vi "snippet get main ui alias names.vi"() -> ()   [LabVIEW 2017]
uses:
  <vilib>/TELLC/CtrlRef/TD UI Control Label-IONames--cluster.ctl
  <vilib>/TELLC/CtrlRef/TD UI Control Label-Alias-IOName--cluster.ctl
  LV_Source/Application/DataTypes/MainUI CtrlRef AliasNames--enum.ctl
panel:
  in  "Ring":u16(ring)
  out "Array":string[](array[string])
  in  "AliasCtrlNames":T1
  in  "UI Control Label Associations":T2={"Controls"=[{"Label"="Application in", "Alias"="", "IOName"=""}, {"Label"="MainTabCtrl", "Alias"="", "IOName"=""}, {"Label"="MoveTowardFast", "Alias"="", "IOName"=""}, {"Label"="MoveToZero", "Alias"="", "IOName"=""}, {"Label"="MoveAwayFast", "Alias"="", "IOName"=""}, {"Label"="MoveToward", "Alias"="", "IOName"=""}, {"Label"="MoveAway", "Alias"="", "IOName"=""}, {"Label"="Safety OK", "Alias"="", "IOName"=""}, {"Label"="SystemError", "Alias"="", "IOName"=""}, {"Label"="Pos Err (cnts)", "Alias"="", "IOName"=""}, {"Label"="MotorPos(in)", "Alias"="", "IOName"=""}, {"Label"="StatusMsg", "Alias"="", "IOName"=""}, {"Label"="Weld Enable", "Alias"="", "IOName"=""}, {"Label"="JoggingTurntable", "Alias"="", "IOName"=""}, {"Label"="JogTurntable", "Alias"="", "IOName"=""}, {"Label"="SeqLoaded", "Alias"="", "IOName"=""}, {"Label"="SeqAborted", "Alias"="", "IOName"=""}, {"Label"="AbortSeq", "Alias"="", "IOName"=""}, {"Label"="MotorCtrlLoop Enable", "Alias"="", "IOName"=""}, {"Label"="Turntable Enable", "Alias"="", "IOName"=""}, {"Label"="SeqRunning", "Alias"="", "IOName"=""}, {"Label"="StartSeq", "Alias"="", "IOName"=""}, {"Label"="Sequence File", "Alias"="", "IOName"=""}, {"Label"="Tab Control", "Alias"="", "IOName"=""}, {"Label"="IgnoreMtrRspnsErr", "Alias"="", "IOName"=""}, {"Label"="AVC ConfigUtility", "Alias"="", "IOName"=""}, {"Label"="SamplingRate", "Alias"="", "IOName"=""}, {"Label"="NumSamples", "Alias"="", "IOName"=""}, {"Label"="UpdateDAQSettings", "Alias"="", "IOName"=""}, {"Label"="DAQ Rd & MtrSP Interval", "Alias"="", "IOName"=""}, {"Label"="WriteLogFile Interval", "Alias"="", "IOName"=""}, {"Label"="DAQDisplay Interval", "Alias"="", "IOName"=""}, {"Label"="DAQEnabled", "Alias"="", "IOName"=""}, {"Label"="DAQEnDis", "Alias"="", "IOName"=""}, {"Label"="LogEnabled", "Alias"="", "IOName"=""}, {"Label"="LogEnDis", "Alias"="", "IOName"=""}, {"Label"="TDMSEnabled", "Alias"="", "IOName"=""}, {"Label"="TDMSEnDis", "Alias"="", "IOName"=""}, {"Label"="PosCtlrSettings", "Alias"="", "IOName"=""}, {"Label"="MotorRspnsErr", "Alias"="", "IOName"=""}, {"Label"="TotalVgain", "Alias"="", "IOName"=""}, {"Label"="Motor SP", "Alias"="", "IOName"=""}, {"Label"="VoltageError", "Alias"="", "IOName"=""}, {"Label"="WeldTime", "Alias"="", "IOName"=""}, {"Label"="voltage fb", "Alias"="", "IOName"=""}, {"Label"="Current SP", "Alias"="", "IOName"=""}, {"Label"="Current fb", "Alias"="", "IOName"=""}, {"Label"="ProcessTime", "Alias"="", "IOName"=""}, {"Label"="AVC Lockout", "Alias"="", "IOName"=""}, {"Label"="In Range?", "Alias"="", "IOName"=""}, {"Label"="VspOffset", "Alias"="", "IOName"=""}, {"Label"="Volts and Current Chart", "Alias"="", "IOName"=""}, {"Label"="GraphEnable", "Alias"="", "IOName"=""}, {"Label"="DAQ Latency", "Alias"="", "IOName"=""}, {"Label"="MotorControlUI", "Alias"="", "IOName"=""}, {"Label"="SeqList", "Alias"="", "IOName"=""}, {"Label"="Step Comment", "Alias"="", "IOName"=""}, {"Label"="Turntable \nSpeed (RPM)", "Alias"="", "IOName"=""}, {"Label"="Process Complete", "Alias"="", "IOName"=""}, {"Label"="Weld Profile Graph", "Alias"="", "IOName"=""}, {"Label"="Weld Current Waveform Chart", "Alias"="", "IOName"=""}, {"Label"="Exit", "Alias"="", "IOName"=""}, {"Label"="LoadSeq", "Alias"="", "IOName"=""}, {"Label"="Exit2", "Alias"="", "IOName"=""}, {"Label"="Get DAQ Data", "Alias"="", "IOName"=""}, {"Label"="DAQ Data", "Alias"="", "IOName"=""}, {"Label"="time stamp", "Alias"="", "IOName"=""}, {"Label"="col 0", "Alias"="", "IOName"=""}, {"Label"="col 1", "Alias"="", "IOName"=""}, {"Label"="col 0 name", "Alias"="", "IOName"=""}, {"Label"="col 1 name", "Alias"="", "IOName"=""}, {"Label"="DI DAQ Data", "Alias"="", "IOName"=""}, {"Label"="Sequence Table", "Alias"="", "IOName"=""}, {"Label"="SeqSteps[]", "Alias"="", "IOName"=""}, {"Label"="SeqFileParams", "Alias"="", "IOName"=""}, {"Label"="Load Seq (debug)", "Alias"="", "IOName"=""}, {"Label"="LoadSeqStatus", "Alias"="", "IOName"=""}, {"Label"="SeqFilePathname", "Alias"="", "IOName"=""}, {"Label"="SeqExecStatus", "Alias"="", "IOName"=""}, {"Label"="LocalSMDirect EvData", "Alias"="", "IOName"=""}, {"Label"="AbortSeq - NonLatchingCtrl", "Alias"="", "IOName"=""}]}
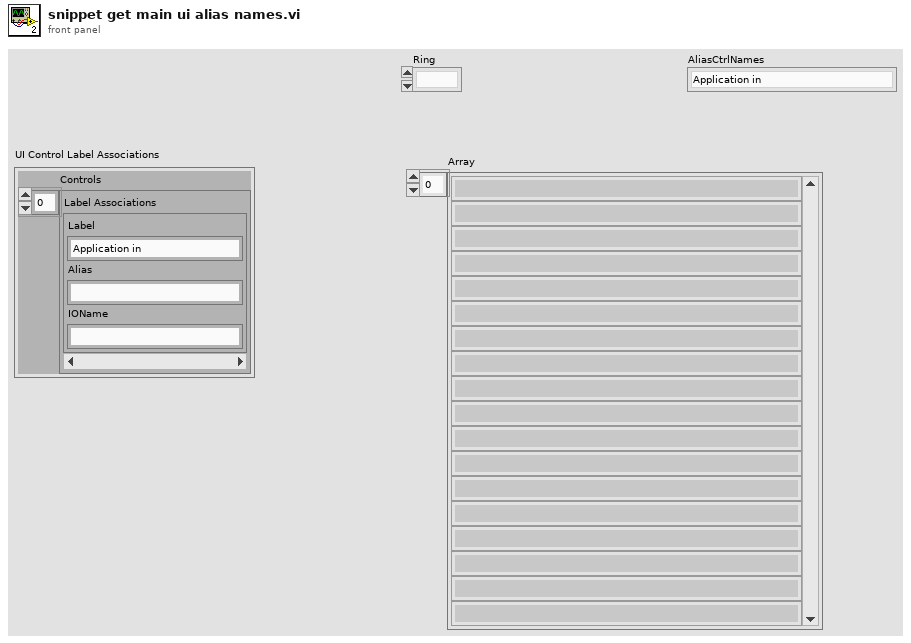
[diagram p1: front panel]
types:
  T1 = typedef "Application.lvclass/MainUI CtrlRef AliasNames--enum.ctl" = enum16{"Application in", "MainTabCtrl", "MoveTowardFast", "MoveToZero", "MoveAwayFast", "MoveToward", "MoveAway", "Safety OK", "SystemError", "Pos Err (cnts)", "MotorPos(in)", "StatusMsg", "Weld Enable", "JoggingTurntable", "JogTurntable", "SeqLoaded", "SeqAborted", "AbortSeq", "MotorCtrlLoop Enable", "Turntable Enable", "SeqRunning", "StartSeq", "Sequence File", "Tab Control", "IgnoreMtrRspnsErr", "AVC ConfigUtility", "SamplingRate", "NumSamples", "UpdateDAQSettings", "DAQ Rd & MtrSP Interval", "WriteLogFile Interval", "DAQDisplay Interval", "DAQEnabled", "DAQEnDis", "LogEnabled", "LogEnDis", "TDMSEnabled", "TDMSEnDis", "PosCtlrSettings", "MotorRspnsErr", "TotalVgain", "Motor SP", "VoltageError", "WeldTime", "voltage fb", "Current SP", "Current fb", "ProcessTime", "AVC Lockout", "In Range?", "VspOffset", "Volts and Current Chart", "GraphEnable", "DAQ Latency", "MotorControlUI", "SeqList", "Step Comment", "Turntable Speed (RPM)", "Process Complete", "Weld Profile Graph", "Weld Current Waveform Chart", "Exit", "LoadSeq", "Exit2", "Get DAQ Data", "DAQ Data", "time stamp", "col 0", "col 1", "col 0 name", "col 1 name", "DI DAQ Data", "Sequence Table", "SeqSteps[]", "SeqFileParams", "Load Seq (debug)", "LoadSeqStatus", "SeqFilePathname", "SeqExecStatus", "LocalSMDirect EvData", "AbortSeq - NonLatchingCtrl"}
  T2 = typedef "TD UI Control Label-IONames--cluster.ctl" = cluster{"Controls":T3[]}
  T3 = typedef "TD UI Control Label-Alias-IOName--cluster.ctl" = cluster{"Label":string, "Alias":string, "IOName":string}
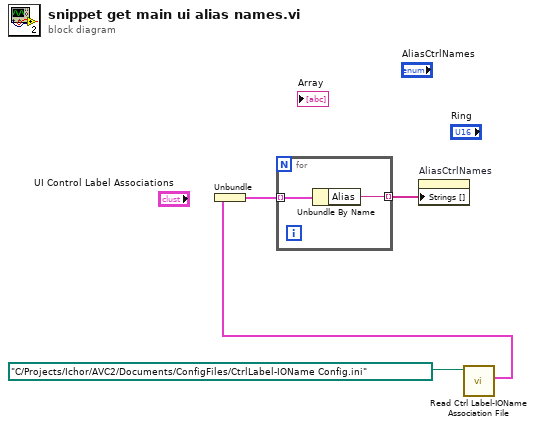
[diagram p0: block diagram]
diagram:
  n1 = call <vilib>:"Read Ctrl Label-IOName Association File.vi"("ConfigFile"=path "C:/Projects/Ichor/AVC2/Documents/ConfigFiles/CtrlLabel-IOName Config.ini") -> ("UI Control Label Associations"=w2:T2)  [unwired: 8 in, 2 out]
  n2 = Unbundle(w2) -> ("Controls"=w4:T3[])
  n3 = for {
    tunnel: w4 -> [w6] mode=indexing
    tunnel: [w5] -> w1 mode=indexing
    n4 = Unbundle By Name(w6) -> ("Alias"=w5:string)
  }
  n5 = property on="AliasCtrlNames" class="Enum (strict)"("Strings []"=w1) -> ()  [unwired: 2 in, 2 out]
